vi "Notify.vi"(5 "Send Notifier Emails?":bool, 6 "Test Matrix":T1, 7 "error in (no error)":errorcluster, 10 "appended path":path) -> (0 "error out":errorcluster)   [LabVIEW 2013]
doc: "modifies test matrix file to indicate that test combination has been completed"
uses:
  Controls/data.ctl
  <vilib>/Utility/file.llb/Write To Spreadsheet File (string).vi
panel:
  out "output array":string[][](array[string])
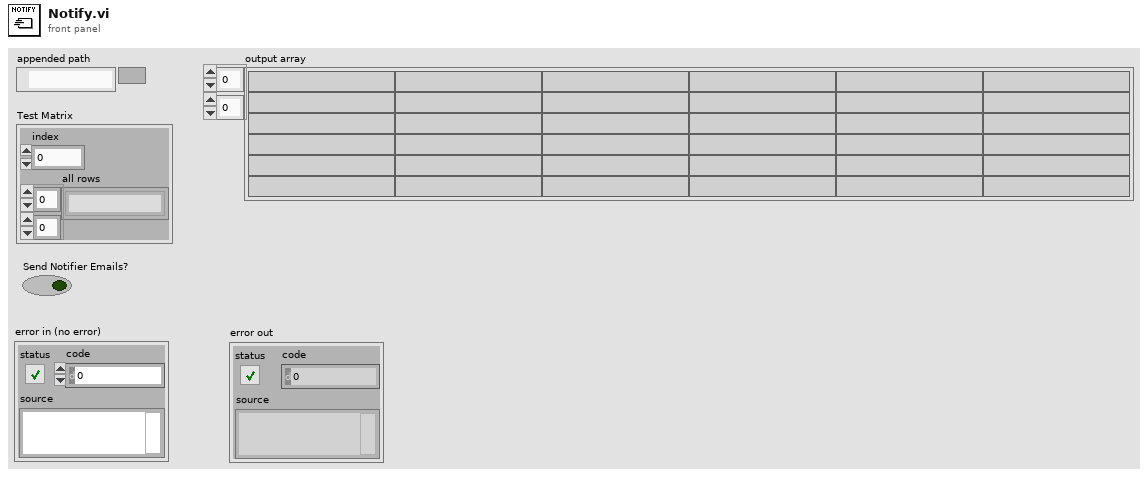
[diagram p1: front panel]
types:
  T1 = typedef "data.ctl" = cluster{"index":i32, "all rows":string[][]}
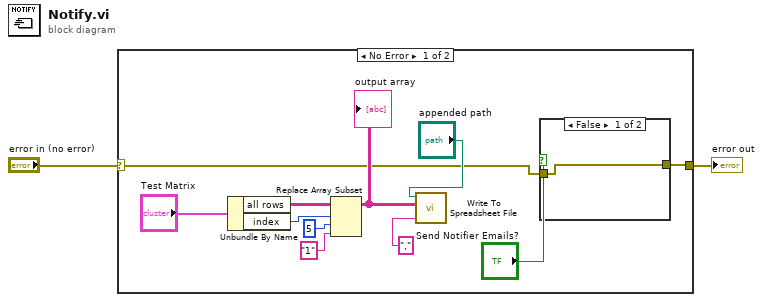
[diagram p0: block diagram]
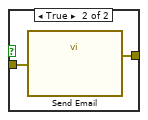
[diagram p2: hidden frame]
diagram:
  n1 = case shown="No Error" "error in (no error)" {
    selector: "error in (no error)" -> [w4 w17]
    tunnel: [w5 w17] -> w1
    frame No Error {
      n2 = Unbundle By Name("Test Matrix") -> ("all rows"=w8:string[][], "index"=w9:i32)
      n3 = Replace Array Subset(array=w8, new element="1" ("new element/subarray"), index (row)=w9, index (col)=5 ("disabled index (col)")) -> (w6:string[][])
      "output array" <- w6
      n4 = call-poly <vilib>:"Write To Spreadsheet File.vi"("delimiter (\\t)"="," ("delimiter (\\t)"), "2D data"=w6, "file path (dialog if empty)"="appended path") -> ()  [unwired: 5 in, 1 out]
      n5 = case shown="False" "Send Notifier Emails?" {
        tunnel: [w14 w16] -> w5
        tunnel: w4 -> [w14 w15]
        frame False {
        }
        frame True {
          n6 = call "Send Email"("error in"=w15) -> ("error out"=w16:errorcluster)  [unwired: 10 in]
        }
      }
    }
    frame Error {
    }
  }
  "error out" <- w1
